vi "ReadDataLine.vi"(8 "error in (no error)":errorcluster, 11 "FTP in":refnum<class "FTP.lvclass">) -> (0 "error out":errorcluster, 2 "Data":string, 3 "FTP out":refnum<class "FTP.lvclass">)   [LabVIEW 2020, in "FTP.lvlib" / "FTP.lvclass"]
uses:
  FTP.lvclass
  FTP.lvclass/FTP.ctl
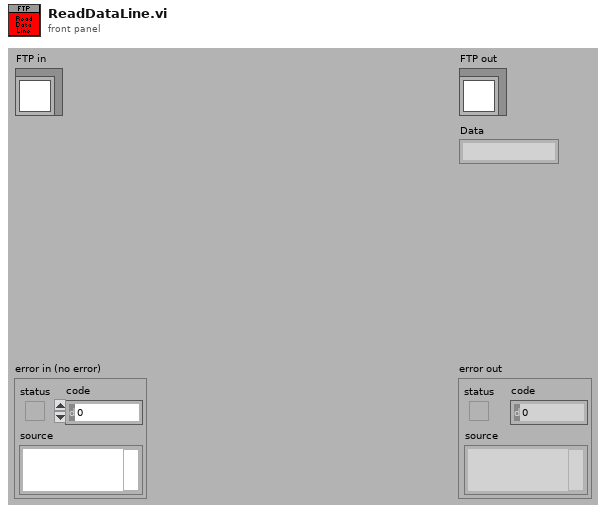
[diagram p1: front panel]
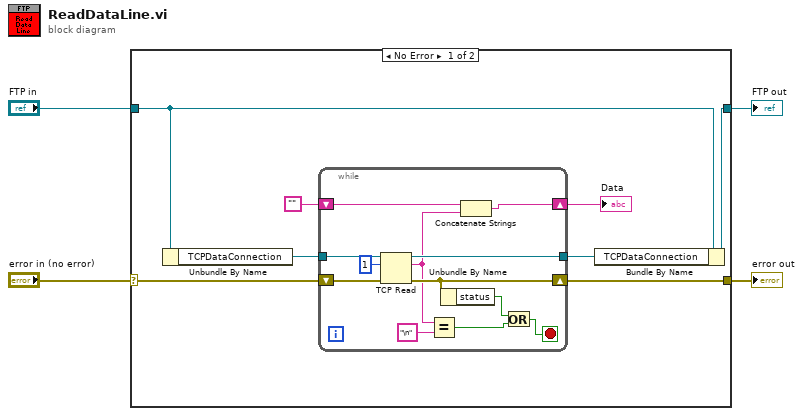
[diagram p0: block diagram]
diagram:
  n1 = case shown="No Error" "error in (no error)" {
    selector: "error in (no error)" -> [w9 w26]
    tunnel: [w8 w26] -> w3
    tunnel: [w7 w25] -> w1
    tunnel: "FTP in" -> [w10 w25]
    frame No Error {
      n2 = Unbundle By Name(w10) -> ("TCPDataConnection"=w11:refnum<k5>)
      n3 = while {
        tunnel: w11 -> [w23]
        tunnel: [w22] -> w6
        shift-right: [w13] -> w5
        shift-left: "" -> [w15]
        shift-right: [w19] -> w8
        shift-left: w9 -> [w24]
        stop <- w18 stop-if-true
        n4 = TCP Read(connection ID=w23, bytes to read=1, error in (no error)=w24) -> (connection ID out=w22:refnum<k5>, data out=w14:string, error out=w19:errorcluster)  [unwired: 2 in]
        n5 = Equal?(x=w14, y="\n") -> (x = y?=w16:bool)
        n6 = Unbundle By Name(w19) -> ("status"=w17:bool)
        n7 = Concatenate Strings(w15, w14) -> (w13:string)
        n8 = Or(x=w17, y=w16) -> (x .or. y?=w18:bool)
      }
      "Data" <- w5
      n9 = Bundle By Name(cluster=w10, "TCPDataConnection"=w6) -> (w7:refnum<class "FTP.lvclass">)
    }
    frame Error {
    }
  }
  "error out" <- w3
  "FTP out" <- w1
